vi "Basic Example.vi"(8 "error in (no error)":errorcluster, 10 "export file path":path, 11 "target in":refnum<k24>) -> (0 "error out":errorcluster)   [LabVIEW 2018]
uses:
  NationalInstruments.VeriStand.SystemDefinitionAPI
  <vilib>/addons/VeriStand Custom Device Scripting APIs/Instrument Addon/Libraries Directory/Protocols.lvlibp/TCP/TCP Settings.ctl
  <vilib>/addons/VeriStand Custom Device Scripting APIs/Instrument Addon/API/TypeDefs/Command Settings.ctl
  <vilib>/NI Veristand/Custom Device API/Custom Device Item Ref.ctl
  <vilib>/addons/VeriStand Custom Device Scripting APIs/Instrument Addon/API/TypeDefs/Padding.ctl
  <vilib>/addons/VeriStand Custom Device Scripting APIs/Instrument Addon/API/TypeDefs/Wait Response Settings.ctl
  <vilib>/addons/VeriStand Custom Device Scripting APIs/Instrument Addon/API/TypeDefs/Linked Channel.ctl
  <vilib>/addons/VeriStand Custom Device Scripting APIs/Instrument Addon/API/Custom Device/TCP Factory.vi
  <vilib>/addons/VeriStand Custom Device Scripting APIs/Instrument Addon/API/Messages/Create Message - Trigger Only.vi
  <vilib>/addons/VeriStand Custom Device Scripting APIs/Instrument Addon/API/Messages/Configure Response - Wait (sec).vi
  <vilib>/addons/VeriStand Custom Device Scripting APIs/Instrument Addon/API/Instrument Addon Scripting API.lvlib
  <vilib>/addons/VeriStand Custom Device Scripting APIs/Instrument Addon/Libraries Directory/Protocols.lvlibp/TCP/TCP.lvclass
  <vilib>/NI VeriStand/Custom Device API/Custom Device API.lvlib
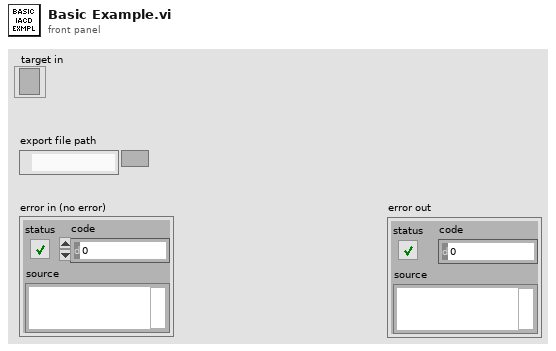
[diagram p1: front panel]
types:
  T1 = typedef "Instrument Addon Scripting API.lvlib/Wait Response Settings.ctl" = cluster{"Response Format":string, "Linked Channels":T2[], "Wait value (sec)":dbl, "Use Wait Channel":bool, "Channel Refnum":T3}
  T2 = typedef "Instrument Addon Scripting API.lvlib/Linked Channel.ctl" = cluster{"Variable Name":string, "Channel Refnum":T3}
  T3 = typedef "Custom Device API.lvlib/Custom Device Item Ref.ctl" = u64
  T4 = typedef "Instrument Addon Scripting API.lvlib/Command Settings.ctl" = cluster{"Command Format":string, "Linked Channels":cluster{"Variable Name":string, "Channel Ref in":T3}[], "Use Padding?":bool, "Padding":T5}
  T5 = typedef "Instrument Addon Scripting API.lvlib/Padding.ctl" = cluster{"Pad Value":u8, "Length":u32}
  T6 = typedef "Protocols.lvlibp/TCP.lvclass/TCP Settings.ctl" = cluster{"IP Address":string, "Port":u16}
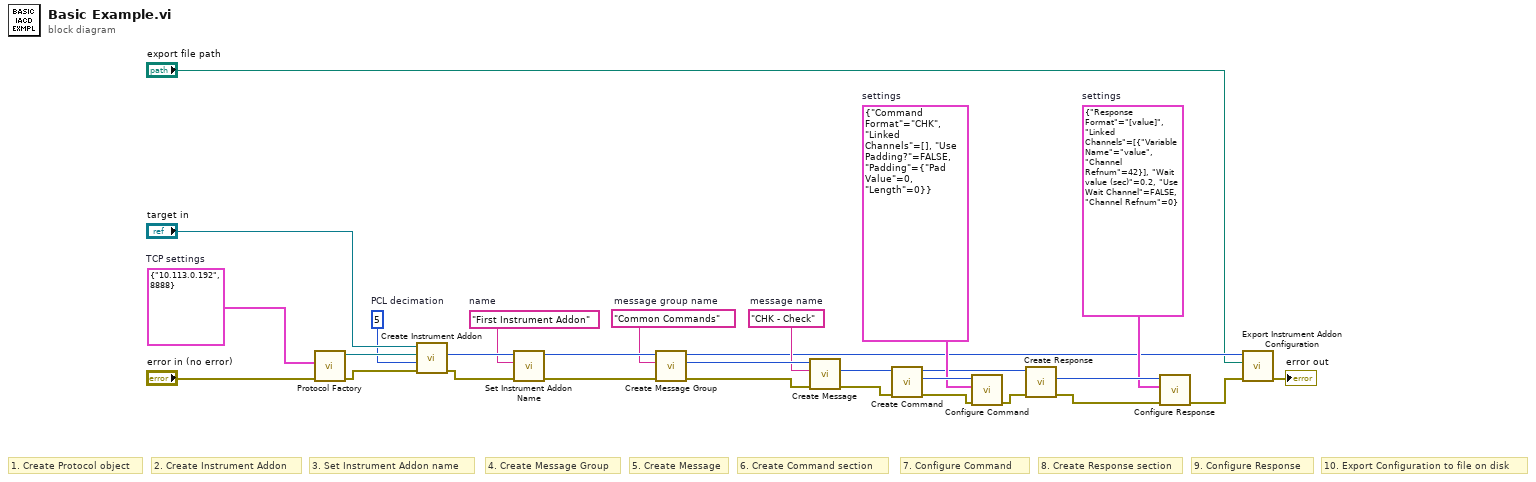
[diagram p0: block diagram]
diagram:
  w5 = T1 {"Response Format"="[value]", "Linked Channels"=[{"Variable Name"="value", "Channel Refnum"=42}], "Wait value (sec)"=0.2, "Use Wait Channel"=FALSE, "Channel Refnum"=0}  # settings
  w11 = T4 {"Command Format"="CHK", "Linked Channels"=[], "Use Padding?"=FALSE, "Padding"={"Pad Value"=0, "Length"=0}}  # settings
  w16 = "CHK - Check"  # message name
  w18 = "Common Commands"  # message group name
  w22 = "First Instrument Addon"  # name
  w24 = u16 5  # PCL decimation
  w29 = T6 {"IP Address"="10.113.0.192", "Port"=8888}  # TCP settings
  # "10. Export Configuration to file on disk"
  # "9. Configure Response"
  # "8. Create Response section"
  # "7. Configure Command"
  # "6. Create Command section"
  # "5. Create Message"
  # "4. Create Message Group"
  # "3. Set Instrument Addon name"
  # "2. Create Instrument Addon"
  # "1. Create Protocol object"
  n1 = call-poly <vilib>:"Protocol Factory.vi"("error in (no error)"="error in (no error)", "TCP settings"=w29) -> ("error out"=w26:errorcluster, "protocol out"=w27:refnum<class "Protocol Parent.lvclass">)  [unwired: 8 in]
  n2 = call <vilib>:"Create Instrument Addon.vi"("error in (no error)"=w26, "PCL decimation"=w24, "protocol in"=w27, "target in"="target in") -> ("error out"=w21:errorcluster, "instrument addon refnum"=w23:T3)  [unwired: 5 in, 1 out]
  n3 = call <vilib>:"Set Instrument Addon Name.vi"("error in (no error)"=w21, "name"=w22, "instrument addon refnum in"=w23) -> ("error out"=w19:errorcluster, "instrument addon refnum out"=w20:T3)  [unwired: 7 in]
  n4 = call <vilib>:"Create Message Group.vi"("error in (no error)"=w19, "message group name"=w18, "instrument addon refnum in"=w20) -> ("error out"=w15:errorcluster, "message group refnum out"=w17:T3, "instrument addon refnum out"=w4:T3)  [unwired: 6 in]
  n5 = call-poly <vilib>:"Create Message.vi"("error in (no error)"=w15, "message name"=w16, "message group refnum in"=w17) -> ("error out"=w13:errorcluster, "message refnum out"=w14:T3)  [unwired: 6 in, 1 out]
  n6 = call <vilib>:"Create Command.vi"("error in"=w13, "message refnum In"=w14) -> ("error out"=w10:errorcluster, "command refnum"=w12:T3, "message refnum out"=w9:T3)  [unwired: 7 in]
  n7 = call <vilib>:"Configure Command.vi"("error in (no error)"=w10, "settings"=w11, "command refnum in"=w12) -> ("error out"=w8:errorcluster)  [unwired: 7 in, 1 out]
  n8 = call <vilib>:"Create Response.vi"("error in (no error)"=w8, "message refnum in"=w9) -> ("error out"=w6:errorcluster, "response refnum"=w7:T3)  [unwired: 7 in, 1 out]
  n9 = call-poly <vilib>:"Configure Response.vi"("error in (no error)"=w6, "settings"=w5, "reponse refnum in"=w7) -> ("error out"=w3:errorcluster)  [unwired: 7 in, 1 out]
  n10 = call <vilib>:"Export Instrument Addon Configuration.vi"("error in (no error)"=w3, "export file path"="export file path", "instrument addon refnum in"=w4) -> ("error out"=→"error out":errorcluster)  [unwired: 7 in, 1 out]
